vi "Repeat Button Press.vi"(0 "GEA2 Reference In":refnum<k24>, 5 "Button":T1=enum."Temp Option ", 7 "Hold Time (s)":dbl format="%#_13g", 9 "How Many Button Presses?":i32=24, 11 "Error Out":errorcluster) -> (4 "GEA2 Reference Out":refnum<k24>, 15 "Error Out":errorcluster)   [LabVIEW 2016]
uses:
  Q:/Common/DLLs/GEA3/GeaCommunication.dll
  Common/DLLs/GEA3/GeaCommunication.dll
  Type Defs/JL_Buttons.ctl
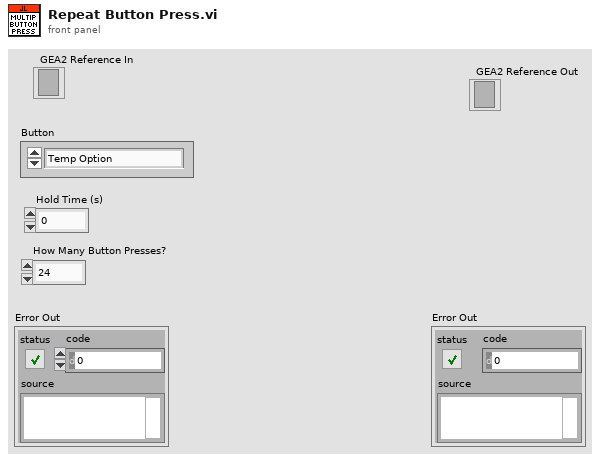
[diagram p1: front panel]
types:
  T1 = typedef "JL_Buttons.ctl" = enum16{"Power", "Start / Pause ", "Temp Option ", "Dryness Level", "Time Option", "Time Increment ", "Time Decrement ", "MyCycle", "eDry ", "Delay", "Extended Tumble", "Control Lock", "Volume/Signal", "Damp Alert / Drum Light", "Unused", "(SW213)", "(SW322)", "Clear / Reset"}
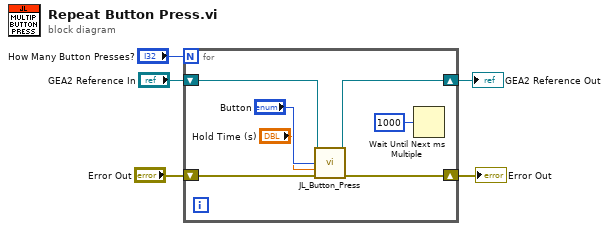
[diagram p0: block diagram]
diagram:
  n1 = for {
    N: "How Many Button Presses?" -> [_]
    shift-right: [w6] -> w4
    shift-left: "Error Out" -> [w12]
    shift-right: [w11] -> w2
    shift-left: "GEA2 Reference In" -> [w10]
    n2 = call "JL_Button_Press.vi"("GEA2 Reference In"=w10, 7:"Button", "Button"="Hold Time (s)", "Error In"=w12) -> ("GEA2 Reference Out"=w11:refnum<k24>, "Error Out"=w6:errorcluster)  [unwired: 10 in]
    n3 = Wait Until Next ms Multiple(millisecond multiple=u32 1000) -> ()  [unwired: 1 out]
  }
  "Error Out" <- w4
  "GEA2 Reference Out" <- w2
